vi "ExponentialFit.vi"() -> ()   [LabVIEW 2014]
uses:
  <vilib>/Waveform/WDTFileIO.llb/Read Waveform from File.vi
panel:
  out "Decay Time (s)":dbl=218.05055115783227
  out "Poisson Fit":waveform(dbl)[](graph)=[{"t0"=timestamp(0 s since 1904-01-01), "dt"=1.0, "Y"=[23.0, 17.0, 26.0, 15.0, 18.0, 27.0, 19.0, 22.0, 32.0, 29.0, 26.0, 30.0, 23.0, 34.0, 24.0, 33.0, 32.0, 22.0, 29.0, 20.0, 35.0, 37.0, 38.0, 27.0, 27.0, 28.0, 32.0, 30.0, 17.0, 33.0, 29.0, 26.0, 23.0, 27.0, 26.0, 36.0, 30.0, 28.0, 25.0, 29.0, 35.0, 29.0, 18.0, 26.0, 36.0, 23.0, 37.0, 29.0, 22.0, 29.0, 26.0, 26.0, 31.0, 29.0, 33.0, 29.0, 25.0, 27.0, 28.0, 18.0, 23.0, 22.0, 21.0, 18.0, 24.0, 23.0, 32.0, 29.0, 27.0, 25.0, 19.0, 22.0, 20.0, 20.0, 28.0, 18.0, 17.0, 22.0, 24.0, 31.0, 23.0, 20.0, 18.0, 24.0, 24.0, 22.0, 21.0, 21.0, 21.0, 25.0, 24.0, 28.0, 28.0, 20.0, 20.0, 35.0, 20.0, 26.0, 18.0, 19.0, 14.0, 15.0, 16.0, 20.0, 21.0, 28.0, 20.0, 24.0, 21.0, 21.0, 24.0, 21.0, 15.0, 22.0, 16.0, 17.0, 17.0, 23.0, 19.0, 17.0, 19.0, 12.0, 19.0, 21.0, 22.0, 25.0, 22.0, 26.0, 24.0, 17.0, 19.0, 15.0, 23.0, 25.0, 17.0, 18.0, 15.0, 17.0, 19.0, 23.0, 13.0, 19.0, 17.0, 17.0, 29.0, 13.0, 16.0, 13.0, 15.0, 14.0, 14.0, 19.0, 31.0, 20.0, 16.0, 19.0, 21.0, 13.0, 11.0, 15.0, 21.0, 18.0, 11.0, 17.0, 11.0, 17.0, 20.0, 11.0, 26.0, 14.0, 17.0, 19.0, 21.0, 13.0, 17.0, 15.0, 16.0, 15.0, 12.0, 20.0, 17.0, 15.0, 12.0, 14.0, 22.0, 15.0, 11.0, 17.0, 16.0, 13.0, 12.0, 13.0, 21.0, 19.0, 19.0, 20.0, 12.0, 24.0, 16.0, 15.0, 22.0, 16.0, 7.0, 13.0, 13.0, 16.0, 26.0, 16.0, 21.0, 18.0, 13.0, 19.0, 15.0, 8.0, 20.0, 11.0, 18.0, 19.0, 21.0, 18.0, 17.0, 11.0, 11.0, 9.0, 12.0, 12.0, 12.0, 18.0, 12.0, 19.0, 18.0, 19.0, 12.0, 16.0, 21.0, 13.0, 13.0, 12.0, 16.0, 8.0, 16.0, 11.0, 15.0, 13.0, 19.0, 17.0, 15.0, 18.0, 18.0, 14.0, 12.0, 7.0, 10.0, 22.0, 15.0, 10.0, 15.0, 19.0, 17.0, 9.0, 11.0, 15.0, 12.0, 21.0, 13.0, 16.0, 14.0, 13.0, 10.0, 11.0, 19.0, 9.0, 12.0, 17.0, 20.0, 7.0, 18.0, 15.0, 13.0, 12.0, 15.0, 14.0, 17.0, 13.0, 12.0, 16.0, 15.0, 22.0, 12.0, 12.0, 9.0, 18.0, 16.0, 13.0, 18.0, 15.0, 12.0, 16.0, 20.0, 11.0]}, {"t0"=timestamp(0 s since 1904-01-01), "dt"=1.0, "Y"=array[300 elements], "attributes"=variant("NI_ChannelName"=variant(string "Best fit"))}]
  in  "Data File":path=path "C:/Users/cnee1/Desktop/week8/decay"
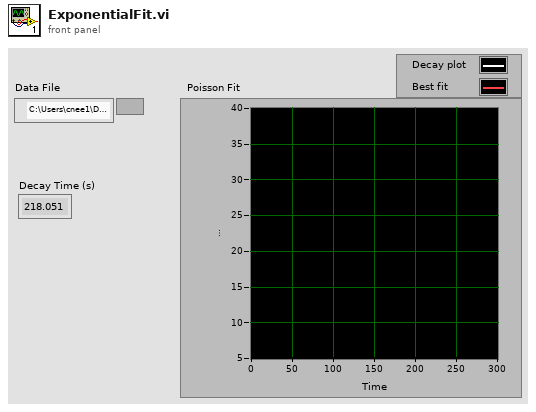
[diagram p1: front panel]
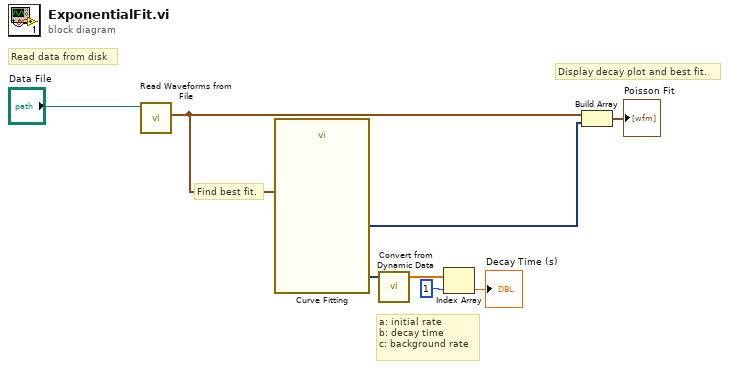
[diagram p0: block diagram]
diagram:
  # "a: initial rate\nb: decay time\nc: background rate"
  # "Find best fit."
  # "Display decay plot and best fit."
  # "Read data from disk"
  n1 = call-poly <vilib>:"Read Waveforms from File.vi"("file path (dialog if empty)"="Data File") -> ("first waveform in record"=w1:waveform(dbl))  [unwired: 5 in, 3 out]
  n2 = call "Curve Fitting"("Signals"=w1) -> ("best fit"=w6:dynamicdata, "non-linear coefficients"=w5:dynamicdata)  [unwired: 6 in, 3 out]
  n3 = call "Convert from Dynamic Data"("Dynamic Data Type"=w5) -> ("Array"=w4:dbl[])  [unwired: 3 in]
  n4 = Index Array(array=w4, index=1) -> (element=→"Decay Time (s)":dbl)
  n5 = Build Array(w1, w6) -> (→"Poisson Fit":waveform(dbl)[])
